vi "Dashboard custom_Ur3_realtimepose.vi"() -> ()   [LabVIEW 2017]
uses:
  C:/Users/IMR Lab/Documents/LabVIEW Data/UniversalRobotsSDK_LABView/LabVIEW/Examples/LabVIEW10/UnderAutomation.UniversalRobots.dll
  UnderAutomation.UniversalRobots.dll
  Global 1.vi
panel:
  out "RY":dbl
  out "RX":dbl
  out "RZ":dbl
  out "Powered on":bool
  in  "Script to execute":string
  in  "Send script":bool
  out "Z":dbl
  out "Y":dbl
  out "X":dbl
  in  "Robot IP(192.168.112.182)":string
  out "Connect error":errorcluster
  in  "Power off":bool
  in  "Power on\nRelease brake":bool
  out "Connected":bool
  out "License state":string
  in  "Connect":bool
  # "1. Connect to the robot"
  # "2. Dashboard"
  # "3. Primary Interface"
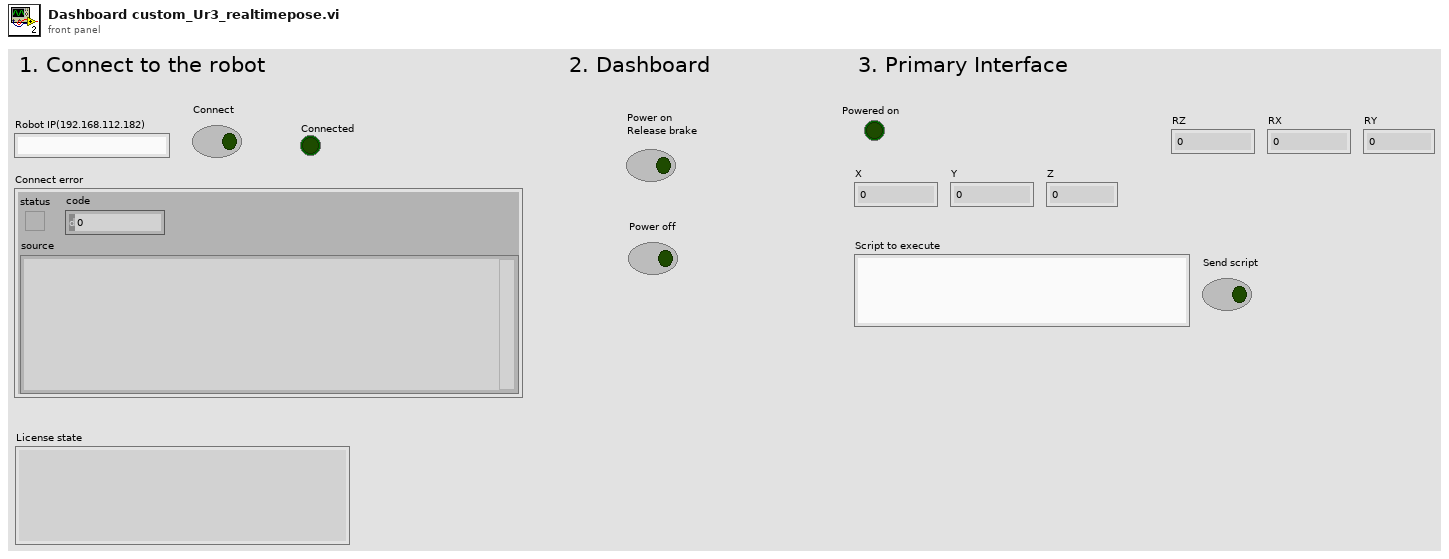
[diagram p1: front panel]
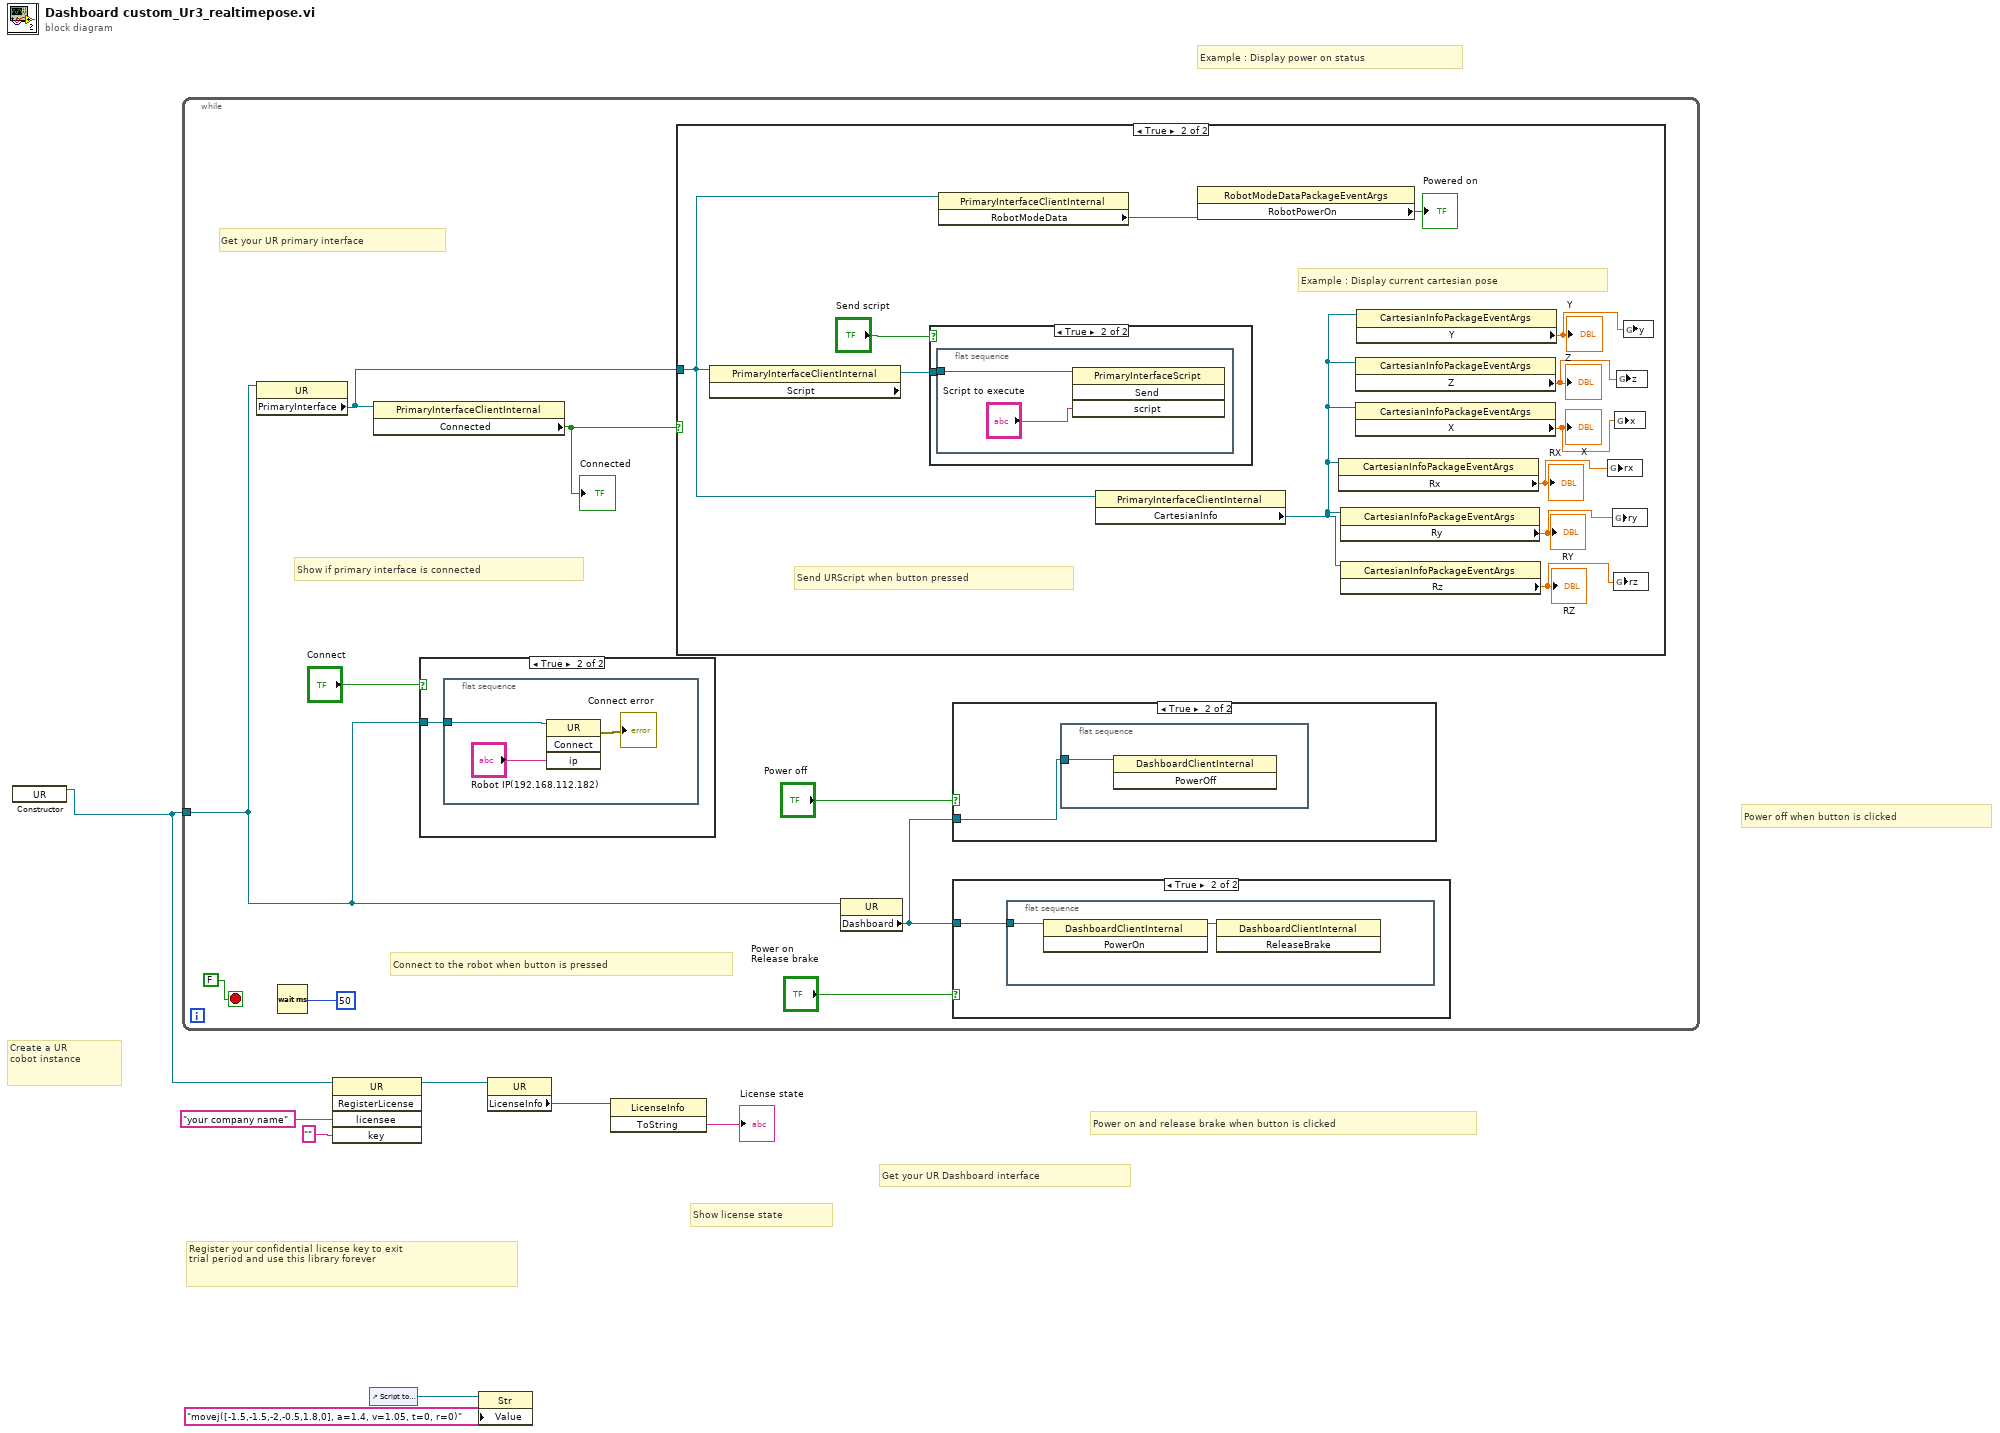
[diagram p0: block diagram]
diagram:
  # "Example : Display power on status"
  # "Create a UR\ncobot instance"
  # "Show license state"
  # "Register your confidential license key to exit\ntrial period and use this library forever"
  # "Power off when button is clicked"
  # "Power on and release brake when button is clicked"
  # "Get your UR Dashboard interface"
  n1 = constructor class="UR"() -> (reference out=w1:refnum<k24>)  [unwired: 3 in, 2 out]
  n2 = while {
    tunnel: w1 -> [w9]
    stop <- FALSE stop-if-true
    # "Connect to the robot when button is pressed"
    # "Show if primary interface is connected"
    # "Get your UR primary interface"
    n3 = property class="UR"(reference=w9) -> ("PrimaryInterface"=w12:refnum<k24>)  [unwired: 1 in, 2 out]
    n4 = Wait (ms)(milliseconds to wait=u32 50) -> ()  [unwired: 1 out]
    n5 = property class="PrimaryInterfaceClientInternal"(reference=w12) -> ("Connected"=w11:bool)  [unwired: 1 in, 2 out]
    "Connected" <- w11
    n6 = case shown="True" "Connect" {
      tunnel: w9 -> [_ w38]
      frame False {
      }
      frame True {
        n7 = flat-sequence {
          tunnel: w38 -> [w40]
          frame #0 {
            n8 = invoke class="UR" method="Connect"(reference=w40, "ip"="Robot IP(192.168.112.182)") -> (error out=→"Connect error":errorcluster)  [unwired: 2 in, 3 out]
          }
        }
      }
    }
    n9 = case shown="True" w11 {
      tunnel: w12 -> [_ w25]
      frame False {
      }
      frame True {
        # "Send URScript when button pressed"
        # "Example : Display current cartesian pose"
        n10 = property class="PrimaryInterfaceClientInternal"(reference=w25) -> ("Script"=w28:refnum<k24>)  [unwired: 1 in, 2 out]
        n11 = case shown="True" "Send script" {
          tunnel: w28 -> [_ w30]
          frame False {
          }
          frame True {
            n12 = flat-sequence {
              tunnel: w30 -> [w32]
              frame #0 {
                n13 = invoke class="PrimaryInterfaceScript" method="Send"(reference=w32, "script"="Script to execute") -> ()  [unwired: 2 in, 4 out]
              }
            }
          }
        }
        n14 = property class="PrimaryInterfaceClientInternal"(reference=w25) -> ("RobotModeData"=w27:refnum<k24>)  [unwired: 1 in, 2 out]
        n15 = property class="PrimaryInterfaceClientInternal"(reference=w25) -> ("CartesianInfo"=w24:refnum<k24>)  [unwired: 1 in, 2 out]
        n16 = property class="RobotModeDataPackageEventArgs"(reference=w27) -> ("RobotPowerOn"=→"Powered on":bool)  [unwired: 1 in, 2 out]
        n17 = property class="CartesianInfoPackageEventArgs"(reference=w24) -> ("Rx"=w20:dbl)  [unwired: 1 in, 2 out]
        "RX" <- w20
        n18 = property class="CartesianInfoPackageEventArgs"(reference=w24) -> ("Ry"=w19:dbl)  [unwired: 1 in, 2 out]
        "RY" <- w19
        n19 = property class="CartesianInfoPackageEventArgs"(reference=w24) -> ("Rz"=w18:dbl)  [unwired: 1 in, 2 out]
        "RZ" <- w18
        n20 = property class="CartesianInfoPackageEventArgs"(reference=w24) -> ("Z"=w22:dbl)  [unwired: 1 in, 2 out]
        "Z" <- w22
        n21 = property class="CartesianInfoPackageEventArgs"(reference=w24) -> ("X"=w21:dbl)  [unwired: 1 in, 2 out]
        "X" <- w21
        n22 = property class="CartesianInfoPackageEventArgs"(reference=w24) -> ("Y"=w23:dbl)  [unwired: 1 in, 2 out]
        "Y" <- w23
        n23 = global write "Global 1.vi" "rx"(w20) -> ()
        n24 = global write "Global 1.vi" "ry"(w19) -> ()
        n25 = global write "Global 1.vi" "rz"(w18) -> ()
        n26 = global write "Global 1.vi" "x"(w21) -> ()
        n27 = global write "Global 1.vi" "z"(w22) -> ()
        n28 = global write "Global 1.vi" "y"(w23) -> ()
      }
    }
    n29 = property class="UR"(reference=w9) -> ("Dashboard"=w13:refnum<k24>)  [unwired: 1 in, 2 out]
    n30 = case shown="True" "Power off" {
      tunnel: w13 -> [_ w33]
      frame False {
      }
      frame True {
        n31 = flat-sequence {
          tunnel: w33 -> [w34]
          frame #0 {
            n32 = invoke class="DashboardClientInternal" method="PowerOff"(reference=w34) -> ()  [unwired: 2 in, 3 out]
          }
        }
      }
    }
    n33 = case shown="True" "Power on\nRelease brake" {
      tunnel: w13 -> [_ w35]
      frame False {
      }
      frame True {
        n34 = flat-sequence {
          tunnel: w35 -> [w37]
          frame #0 {
            n35 = invoke class="DashboardClientInternal" method="PowerOn"(reference=w37) -> (reference out=w36:refnum<k24>)  [unwired: 2 in, 2 out]
            n36 = invoke class="DashboardClientInternal" method="ReleaseBrake"(reference=w36) -> ()  [unwired: 2 in, 3 out]
          }
        }
      }
    }
  }
  n37 = invoke class="UR" method="RegisterLicense"(reference=w1, "licensee"="your company name", "key"="") -> (reference out=w5:refnum<k24>)  [unwired: 2 in, 4 out]
  n38 = control-ref of="Script to execute"() -> (w3:refnum<vi>)
  n39 = property class="Str"(reference=w3, "Value"="movej([-1.5,-1.5,-2,-0.5,1.8,0], a=1.4, v=1.05, t=0, r=0)") -> ()  [unwired: 1 in, 2 out]
  n40 = property class="UR"(reference=w5) -> ("LicenseInfo"=w4:refnum<k24>)  [unwired: 1 in, 2 out]
  n41 = invoke class="LicenseInfo" method="ToString"(reference=w4) -> ("ToString"=→"License state":string)  [unwired: 2 in, 2 out]
